vi "RemoveByType.vi"(7 "LabVIEW Object Type":refnum<class>, 8 "error in (no error)":errorcluster, 11 "CollectionByRef in":refnum<class "CollectionByRef.lvclass">) -> (0 "error out":errorcluster, 1 "found":bool, 2 "LabVIEW Objects":refnum<class>[](array[class]), 3 "CollectionByRef out":refnum<class "CollectionByRef.lvclass">)   [LabVIEW 2021, in "Collection.lvlib" / "CollectionByRef.lvclass"]
uses:
  CollectionByRef.lvclass
  CollectionByRef.lvclass/CollectionByRef.ctl
  CollectionByValue/CollectionByValue.lvclass
panel:
  out "Removed Names":string[](array[string])
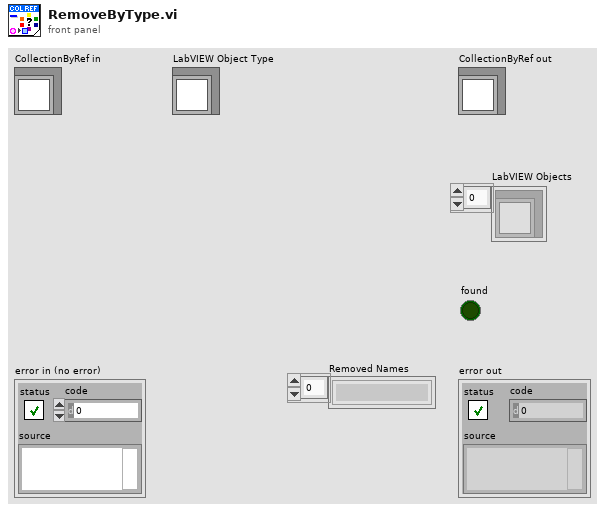
[diagram p1: front panel]
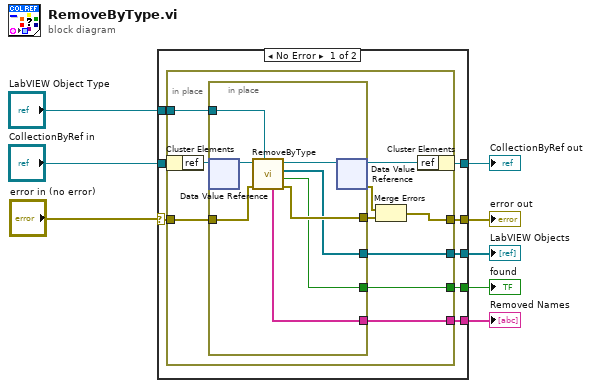
[diagram p0: block diagram]
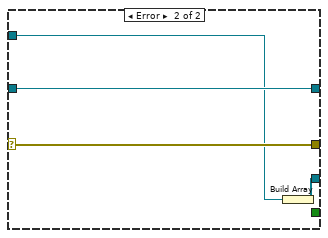
[diagram p2: hidden frame]
diagram:
  n1 = case shown="No Error" "error in (no error)" {
    selector: "error in (no error)" -> [w14 w38]
    tunnel: [w13 w38] -> w6
    tunnel: [w15 w37] -> w7
    tunnel: "CollectionByRef in" -> [w16 w37]
    tunnel: "LabVIEW Object Type" -> [w12 w36]
    tunnel: [w11 w35] -> w3
    tunnel: [w10 _] -> w2
    tunnel: [w9 _] -> w1
    frame No Error {
      n2 = in-place {
        in-place-border: w14 -> [w24]
        in-place-border: [w21] -> w13
        in-place-border: w12 -> [w20]
        in-place-border: [w19] -> w11
        in-place-border: [w18] -> w10
        in-place-border: [w17] -> w9
        n3 = in-place-cluster #1(w16) -> ("ref"=w25:refnum<data-value>)
        n4 = in-place {
          in-place-border: w24 -> [w32]
          in-place-border: [w31] -> w22
          in-place-border: w20 -> [w30]
          in-place-border: [w29] -> w19
          in-place-border: [w28] -> w18
          in-place-border: [w27] -> w17
          n5 = in-place-dvr #2(w25) -> (w34:refnum<class "CollectionByValue.lvclass">)  [unwired: 1 out]
          n6 = call "RemoveByType.vi"("LabVIEW Object Type"=w30, "error in (no error)"=w32, "Collection in"=w34) -> ("error out"=w31:errorcluster, "Found"=w28:bool, "Removed Objects"=w29:refnum<class>[], "Collection out"=w33:refnum<class "CollectionByValue.lvclass">, "Removed Names"=w27:string[])  [unwired: 4 in]
          n7 = in-place-dvr #2(w33) -> (w26:refnum<data-value>, w23:errorcluster)
        }
        n8 = Merge Errors(w23, w22) -> (w21:errorcluster)
        n9 = in-place-cluster #1("ref"=w26) -> (w15:refnum<class "CollectionByRef.lvclass">)
      }
    }
    frame Error {
      n10 = Build Array(w36) -> (w35:refnum<class>[])
    }
  }
  "error out" <- w6
  "CollectionByRef out" <- w7
  "LabVIEW Objects" <- w3
  "found" <- w2
  "Removed Names" <- w1
